vi "Stop Core.vi"(10 "final error code":i32, 11 "Topic In":refnum<class "Topic.lvclass">) -> (3 "Topic Out":refnum<class "Topic.lvclass">)   [LabVIEW 2019, in "Mediator.lvlib" / "Topic.lvclass"]
doc: "(<B>Filename</B>: Actor Framework.lvlib:Actor.lvclass:Stop Core.vi)\n\nDefines what the actor does before it stops. Use the <B>final error code</B> input to determine whether the actor shut down in response to an error.\n\nBy default, this method does nothing. A descendant class may override it to define behavior, such as shutting down any processes the actor initiated in its override of the Actor Core method."
uses:
  <vilib>/gpm_packages/@cs/mva-core/Source/Mediator/Topic/Topic.lvclass
  <vilib>/ActorFramework/Actor/Actor.lvclass
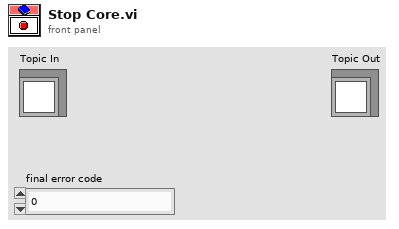
[diagram p1: front panel]
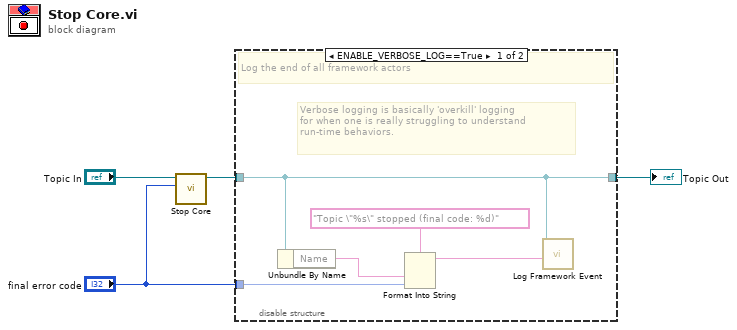
[diagram p0: block diagram]
diagram:
  n1 = call-parent "Stop Core.vi"("final error code"="final error code", "Actor in"="Topic In") -> ("Actor out"=w3:refnum<class "Topic.lvclass">)  [unwired: 9 in]
  n2 = disable-structure shown="ENABLE_VERBOSE_LOG==True" {
    disable-tunnel: w3 -> [w6 w10]
    disable-tunnel: [w6 w10] -> w2
    disable-tunnel: "final error code" -> [w9 _]
    frame condition #0 {
      # "Verbose logging is basically 'overkill' logging\nfor when one is really struggling to understand\nrun-time behaviors."
      # "Log the end of all framework actors"
      n3 = Unbundle By Name(w6) -> ("Name"=w5:string)
      n4 = Format Into String(format string="Topic \"%s\" stopped (final code: %d)", w5, w9) -> (resulting string=w7:string)  [unwired: 2 in, 1 out]
      n5 = call <vilib>:"Log Framework Event.vi"("Data To Log"=w7, "Topic In"=w6) -> ()  [unwired: 9 in, 1 out]
    }
    frame condition #1 (active) {
      # "Remove all logging from this method at compile time"
    }
  }
  "Topic Out" <- w2
